vi "PC_Corner_Detection (DONE).vi"(8 "Error In":errorcluster, 9 "Puck and Player Position":T1, 11 "Image In":T2) -> (0 "Error Out":errorcluster, 1 "Puck and Player Position (Through)":T1, 2 "Table Walls":sgl[](array[numeric]), 3 "Image Out":T2)   [LabVIEW 2017]
uses:
  <vilib>/vision/Image Controls.llb/IMAQ Image.ctl
  <vilib>/vision/Measure.llb/Edge Options.ctl
  <vilib>/vision/Measure.llb/Edge Polarity.ctl
  <vilib>/vision/NI_Vision_Development_Module.lvlib
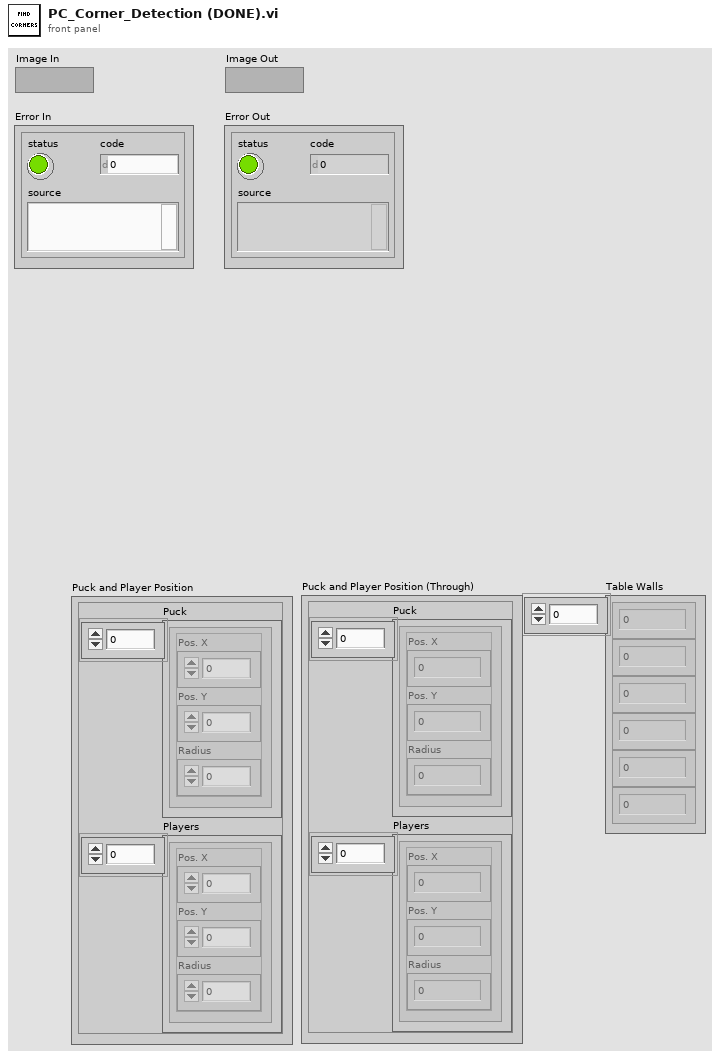
[diagram p1: front panel]
types:
  T1 = cluster{"Puck":cluster{"Pos. X":i32, "Pos. Y":i32, "Radius":i32}[], "Players":cluster{"Pos. X":i32, "Pos. Y":i32, "Radius":i32}[]}
  T2 = typedef "IMAQ Image.ctl" = refnum<image>
  T3 = typedef "Edge Options.ctl" = cluster{"Edge Polarity":T4, "Kernel Size":u32, "Width":u32, "Minimum Edge Strength":sgl, "Interpolation Type":enum32{"Zero Order", "Bilinear", "Quadratic", "Cubic", "Bilinear Fixed"}, "Data Processing Method":enum32{"Average", "Median"}}
  T4 = typedef "Edge Polarity.ctl" = u32
  T5 = cluster{"Search Direction":u32, "Edge Options":T3, "Show Search Area":bool, "Show Search Lines":bool, "Show Edges Found":bool, "Show Result":bool, "Search Area Color":u32, "Search Lines Color":u32, "Edge Locations Color":u32, "Result Color":u32, "Overlay Group Name":string}
  T6 = typedef "ROI Descriptor" = cluster{"Global Rectangle":i32[], "Contours":cluster{"ID":enum32{"External", "Internal"}, "Type":u32, "Coordinates":i32[]}[]}
  T7 = cluster{"Point1 (Pixels)":cluster{"X":sgl, "Y":sgl}, "Point2 (Pixels)":cluster{"X":sgl, "Y":sgl}, "Point1 (Real-World)":cluster{"X":sgl, "Y":sgl}, "Point2 (Real-World)":cluster{"X":sgl, "Y":sgl}, "Angle (Pixel)":dbl, "Angle (Real-World)":dbl, "Score":dbl, "Straightness":dbl, "Average SNR (db)":dbl, "Calibration Valid":bool}[]
  T8 = cluster{"Point1 (Pixels)":cluster{"X":sgl, "Y":sgl}, "Point2 (Pixels)":cluster{"X":sgl, "Y":sgl}, "Point1 (Real-World)":cluster{"X":sgl, "Y":sgl}, "Point2 (Real-World)":cluster{"X":sgl, "Y":sgl}, "Angle (Pixel)":dbl, "Angle (Real-World)":dbl, "Score":dbl, "Straightness":dbl, "Average SNR (db)":dbl, "Calibration Valid":bool}
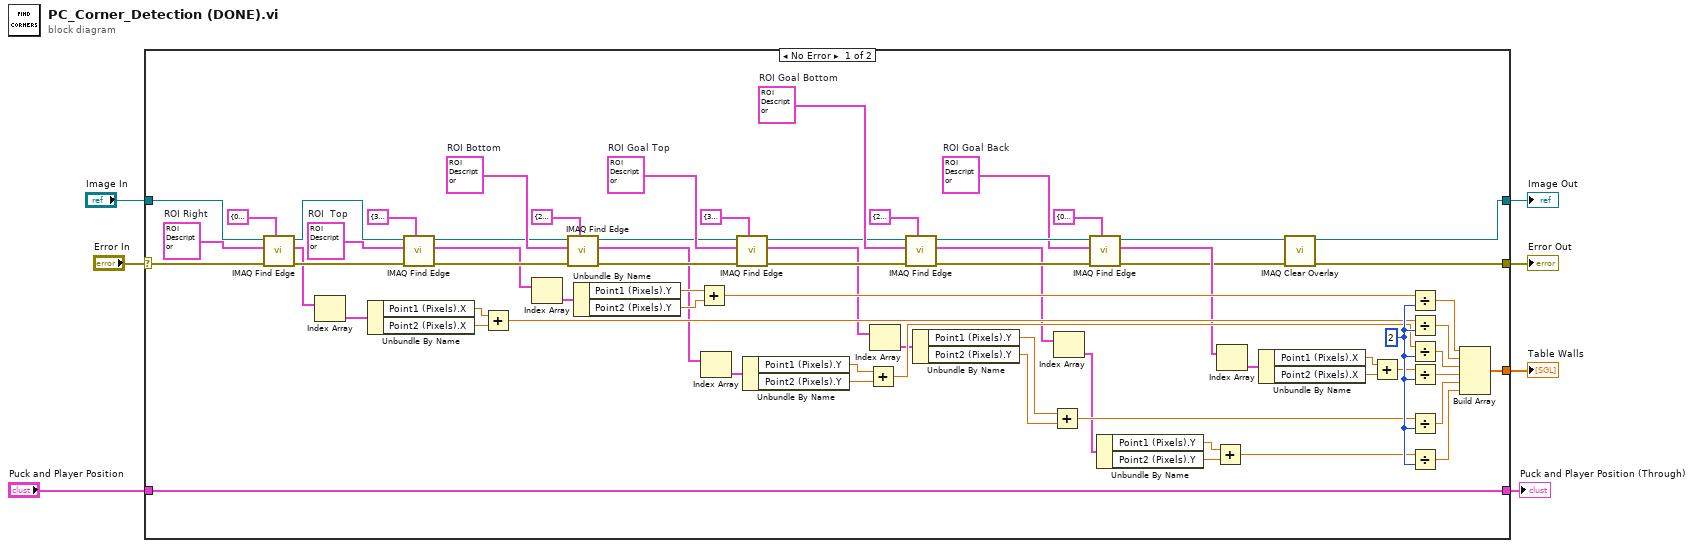
[diagram p0: block diagram]
diagram:
  n1 = case shown="No Error" "Error In" {
    selector: "Error In" -> [w55 w77]
    tunnel: [w10 w76] -> w7
    tunnel: [w11 w77] -> w6
    tunnel: "Image In" -> [w58 w76]
    tunnel: [w13 _] -> w3
    tunnel: "Puck and Player Position" -> [w8 w75]
    tunnel: [w8 w75] -> w1
    frame No Error {
      w50 = 2
      w51 = T6 {"Global Rectangle"=[1206, 358, 1272, 701], "Contours"=[{"ID"=enum."External", "Type"=12, "Coordinates"=[1206, 358, 1272, 701, 0]}]}  # ROI Goal Back
      w72 = T6 {"Global Rectangle"=[1073, 499, 1264, 807], "Contours"=[{"ID"=enum."External", "Type"=12, "Coordinates"=[1073, 499, 1264, 807, 0]}]}  # ROI Goal Bottom
      w71 = T6 {"Global Rectangle"=[1070, 250, 1261, 551], "Contours"=[{"ID"=enum."External", "Type"=12, "Coordinates"=[1070, 250, 1261, 551, 0]}]}  # ROI Goal Top
      w66 = T6 {"Global Rectangle"=[192, 945, 1171, 1031], "Contours"=[{"ID"=enum."External", "Type"=12, "Coordinates"=[192, 945, 1171, 1031, 0]}]}  # ROI Bottom
      w56 = T6 {"Global Rectangle"=[1064, 32, 1202, 1035], "Contours"=[{"ID"=enum."External", "Type"=12, "Coordinates"=[1064, 32, 1202, 1035, 0]}]}  # ROI Right
      w61 = T6 {"Global Rectangle"=[154, 29, 1187, 147], "Contours"=[{"ID"=enum."External", "Type"=12, "Coordinates"=[154, 29, 1187, 147, 0]}]}  # ROI  Top
      n2 = call "IMAQ Find Edge"("Options"=T5 {"Search Direction"=0, "Edge Options"={"Edge Polarity"=0, "Kernel Size"=3, "Width"=3, "Minimum Edge Strength"=10.0, "Interpolation Type"=enum."Bilinear Fixed", "Data Processing Method"=enum."Median"}, "Show Search Area"=FALSE, "Show Search Lines"=FALSE, "Show Edges Found"=FALSE, "Show Result"=TRUE, "Search Area Color"=65280, "Search Lines Color"=255, "Edge Locations Color"=16776960, "Result Color"=16711680, "Overlay Group Name"=""}, "error in (no error)"=w55, "ROI Descriptor"=w56, "Image"=w58) -> ("error out"=w60:errorcluster, "Straight Edges"=w43:T7, "Image Out"=w62:T2)  [unwired: 4 in, 1 out]
      n3 = Index Array(array=w43) -> (element=w42:T8)  [unwired: 1 in]
      n4 = Unbundle By Name(w42) -> ("Point1 (Pixels).X"=w41:sgl, "Point2 (Pixels).X"=w40:sgl)
      n5 = call "IMAQ Find Edge"("Options"=T5 {"Search Direction"=3, "Edge Options"={"Edge Polarity"=0, "Kernel Size"=3, "Width"=3, "Minimum Edge Strength"=10.0, "Interpolation Type"=enum."Bilinear Fixed", "Data Processing Method"=enum."Median"}, "Show Search Area"=FALSE, "Show Search Lines"=FALSE, "Show Edges Found"=FALSE, "Show Result"=TRUE, "Search Area Color"=65280, "Search Lines Color"=255, "Edge Locations Color"=16776960, "Result Color"=16711680, "Overlay Group Name"=""}, "error in (no error)"=w60, "ROI Descriptor"=w61, "Image"=w62) -> ("error out"=w64:errorcluster, "Straight Edges"=w38:T7, "Image Out"=w65:T2)  [unwired: 4 in, 1 out]
      n6 = Add(x=w41, y=w40) -> (x+y=w48:sgl)
      n7 = Index Array(array=w38) -> (element=w39:T8)  [unwired: 1 in]
      n8 = call "IMAQ Find Edge"("Options"=T5 {"Search Direction"=2, "Edge Options"={"Edge Polarity"=0, "Kernel Size"=3, "Width"=3, "Minimum Edge Strength"=10.0, "Interpolation Type"=enum."Bilinear Fixed", "Data Processing Method"=enum."Median"}, "Show Search Area"=FALSE, "Show Search Lines"=FALSE, "Show Edges Found"=FALSE, "Show Result"=TRUE, "Search Area Color"=65280, "Search Lines Color"=255, "Edge Locations Color"=16776960, "Result Color"=16711680, "Overlay Group Name"=""}, "error in (no error)"=w64, "ROI Descriptor"=w66, "Image"=w65) -> ("error out"=w68:errorcluster, "Straight Edges"=w35:T7, "Image Out"=w69:T2)  [unwired: 4 in, 1 out]
      n9 = Unbundle By Name(w39) -> ("Point1 (Pixels).Y"=w37:sgl, "Point2 (Pixels).Y"=w36:sgl)
      n10 = Add(x=w37, y=w36) -> (x+y=w49:sgl)
      n11 = Index Array(array=w35) -> (element=w34:T8)  [unwired: 1 in]
      n12 = call "IMAQ Find Edge"("Options"=T5 {"Search Direction"=3, "Edge Options"={"Edge Polarity"=0, "Kernel Size"=3, "Width"=3, "Minimum Edge Strength"=50.0, "Interpolation Type"=enum."Bilinear Fixed", "Data Processing Method"=enum."Median"}, "Show Search Area"=FALSE, "Show Search Lines"=FALSE, "Show Edges Found"=FALSE, "Show Result"=TRUE, "Search Area Color"=65280, "Search Lines Color"=255, "Edge Locations Color"=16776960, "Result Color"=16711680, "Overlay Group Name"=""} ("Options 2"), "error in (no error)"=w68, "ROI Descriptor"=w71, "Image"=w69) -> ("error out"=w67:errorcluster, "Straight Edges"=w31:T7, "Image Out"=w70:T2)  [unwired: 4 in, 1 out]
      n13 = Unbundle By Name(w34) -> ("Point1 (Pixels).Y"=w33:sgl, "Point2 (Pixels).Y"=w32:sgl)
      n14 = Add(x=w33, y=w32) -> (x+y=w46:sgl)
      n15 = Index Array(array=w31) -> (element=w30:T8)  [unwired: 1 in]
      n16 = call "IMAQ Find Edge"("Options"=T5 {"Search Direction"=2, "Edge Options"={"Edge Polarity"=0, "Kernel Size"=3, "Width"=3, "Minimum Edge Strength"=50.0, "Interpolation Type"=enum."Bilinear Fixed", "Data Processing Method"=enum."Median"}, "Show Search Area"=FALSE, "Show Search Lines"=FALSE, "Show Edges Found"=FALSE, "Show Result"=TRUE, "Search Area Color"=65280, "Search Lines Color"=255, "Edge Locations Color"=16776960, "Result Color"=16711680, "Overlay Group Name"=""} ("Options 2"), "error in (no error)"=w67, "ROI Descriptor"=w72, "Image"=w70) -> ("error out"=w54:errorcluster, "Straight Edges"=w27:T7, "Image Out"=w53:T2)  [unwired: 4 in, 1 out]
      n17 = Unbundle By Name(w30) -> ("Point1 (Pixels).Y"=w29:sgl, "Point2 (Pixels).Y"=w28:sgl)
      n18 = Add(x=w29, y=w28) -> (x+y=w47:sgl)
      n19 = Index Array(array=w27) -> (element=w26:T8)  [unwired: 1 in]
      n20 = call "IMAQ Find Edge"("Options"=T5 {"Search Direction"=0, "Edge Options"={"Edge Polarity"=0, "Kernel Size"=3, "Width"=3, "Minimum Edge Strength"=50.0, "Interpolation Type"=enum."Bilinear Fixed", "Data Processing Method"=enum."Median"}, "Show Search Area"=FALSE, "Show Search Lines"=FALSE, "Show Edges Found"=FALSE, "Show Result"=TRUE, "Search Area Color"=65280, "Search Lines Color"=255, "Edge Locations Color"=16776960, "Result Color"=16711680, "Overlay Group Name"=""} ("Options 2"), "error in (no error)"=w54, "ROI Descriptor"=w51, "Image"=w53) -> ("error out"=w12:errorcluster, "Straight Edges"=w23:T7, "Image Out"=w9:T2)  [unwired: 4 in, 1 out]
      n21 = Unbundle By Name(w26) -> ("Point1 (Pixels).Y"=w25:sgl, "Point2 (Pixels).Y"=w24:sgl)
      n22 = Add(x=w25, y=w24) -> (x+y=w45:sgl)
      n23 = Index Array(array=w23) -> (element=w22:T8)  [unwired: 1 in]
      n24 = Unbundle By Name(w22) -> ("Point1 (Pixels).X"=w21:sgl, "Point2 (Pixels).X"=w20:sgl)
      n25 = call "IMAQ Clear Overlay"("error in (no error)"=w12, "Image"=w9) -> ("error out"=w11:errorcluster, "Image Out"=w10:T2)  [unwired: 8 in]
      n26 = Add(x=w21, y=w20) -> (x+y=w44:sgl)
      n27 = Divide(x=w49, y=w50) -> (x/y=w19:sgl)
      n28 = Divide(x=w48, y=w50) -> (x/y=w18:sgl)
      n29 = Divide(x=w46, y=w50) -> (x/y=w17:sgl)
      n30 = Divide(x=w44, y=w50) -> (x/y=w16:sgl)
      n31 = Divide(x=w47, y=w50) -> (x/y=w15:sgl)
      n32 = Divide(x=w45, y=w50) -> (x/y=w14:sgl)
      n33 = Build Array(w19, w18, w17, w16, w15, w14) -> (w13:sgl[])
    }
    frame Error {
    }
  }
  "Image Out" <- w7
  "Error Out" <- w6
  "Table Walls" <- w3
  "Puck and Player Position (Through)" <- w1
